vi "MCP2221_OpenBySN.vi"(11 "serialNumber":string) -> (0 "error out":errorcluster, 1 "handle out":i32)   [LabVIEW 2025]
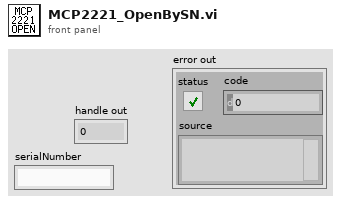
[diagram p1: front panel]
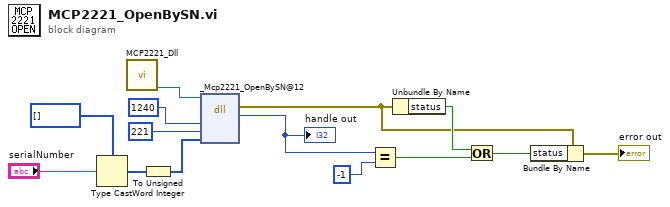
[diagram p0: block diagram]
diagram:
  n1 = Type Cast(type=u8[] [], x="serialNumber") -> (*(type *) &x=w2:u8[])
  n2 = call "MCP2221_Dll.vi"() -> ("dll path"=w12:path)  [unwired: 11 in]
  n3 = To Unsigned Word Integer(number=w2) -> (unsigned 16bit integer=w1:u16[])
  n4 = dll-call lib="?" fn="_Mcp2221_OpenBySN@12"(path in=w12, "vid"=u32 1240, "pid"=u32 221, "serialNo"=w1) -> (error out=w6:errorcluster, "return type"=w11:i32)  [unwired: 5 in, 1 out]
  "handle out" <- w11
  n5 = Equal?(x=w11, y=-1) -> (x = y?=w9:bool)
  n6 = Unbundle By Name(w6) -> ("status"=w10:bool)
  n7 = Or(x=w10, y=w9) -> (x .or. y?=w7:bool)
  n8 = Bundle By Name(cluster=w6, "status"=w7) -> (→"error out":errorcluster)
